vi "playing with images 2.vi"() -> ()   [LabVIEW 2018]
panel:
  in  "Numeric 2":dbl
  in  "Numeric":dbl
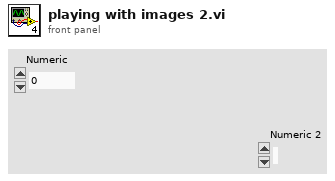
[diagram p1: front panel]
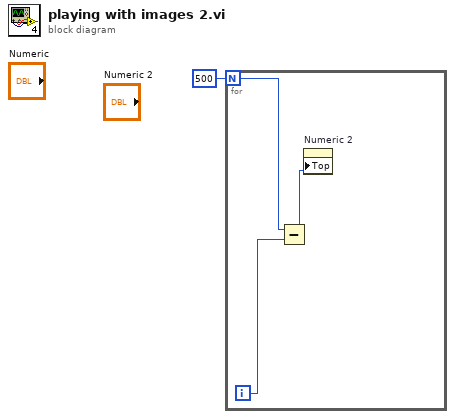
[diagram p0: block diagram]
diagram:
  n1 = for {
    N: 500 -> [w4]
    i -> [w3]
    n2 = Subtract(x=w4, y=w3) -> (x-y=w2:i32)
    n3 = property on="Numeric 2" class="DigNum (strict)"("Top"=w2) -> ()  [unwired: 2 in, 2 out]
  }
